vi "SVT Limit Testing.vi"   [LabVIEW 2017]
doc: "Performs limit testing on waveforms, spectra, XY data, identified peaks, or scalar measurements. You can wire <B>output values</B> to a graph to view the limits, signal, and failures. You can use this polymorphic VI to perform limit testing of a waveform, a waveform with scalar limits, a spectrum, a spectrum with scalar limits, XY data, XY data with scalar limits, peaks, peaks with scalar limits, or a scalar value. The data type you wire to the <B>signal in</B> input determines the polymorphic instance to use."
uses:
  <vilib>/addons/Sound and Vibration/svt_Limit Test/SoundVib_LimitTest.lvlib
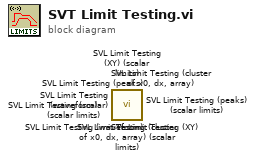
[diagram p0: block diagram]
diagram:
  n1 = call <vilib>:"SVL Limit Testing (cluster of x0, dx, array) (scalar limits).vi"() -> ()  [unwired: 8 in, 4 out]
  n2 = call <vilib>:"SVL Limit Testing (cluster of x0, dx, array).vi"() -> ()  [unwired: 8 in, 4 out]
  n3 = call <vilib>:"SVL Limit Testing (scalar).vi"() -> ()  [unwired: 9 in, 3 out]
  n4 = call <vilib>:"SVL Limit Testing (peaks) (scalar limits).vi"() -> ()  [unwired: 8 in, 4 out]
  n5 = call <vilib>:"SVL Limit Testing (peaks).vi"() -> ()  [unwired: 8 in, 4 out]
  n6 = call <vilib>:"SVL Limit Testing (XY) (scalar limits).vi"() -> ()  [unwired: 8 in, 4 out]
  n7 = call <vilib>:"SVL Limit Testing (XY).vi"() -> ()  [unwired: 8 in, 4 out]
  n8 = call <vilib>:"SVL Limit Testing (waveform) (scalar limits).vi"() -> ()  [unwired: 8 in, 4 out]
  n9 = call <vilib>:"SVL Limit Testing (waveform).vi"() -> ()  [unwired: 8 in, 4 out]
